vi "WriteOutSSH.vi"(11 "Write":string) -> (3 "text read":string)   [LabVIEW 2019]
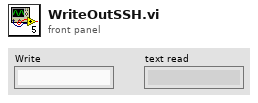
[diagram p1: front panel]
types:
  T1 = enum16{"init", "read", "write", "close", "wait", "reply"}
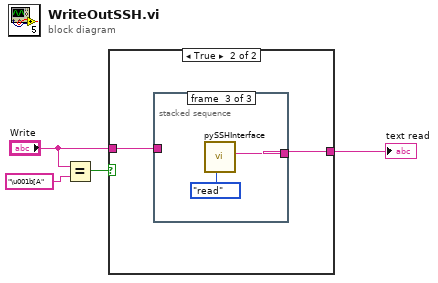
[diagram p0: block diagram]
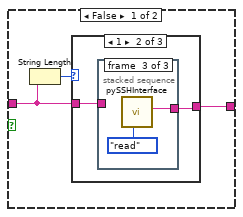
[diagram p2: hidden frame]
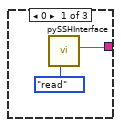
[diagram p3: hidden frame]
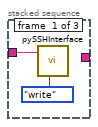
[diagram p4: hidden frame]
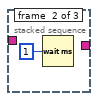
[diagram p5: hidden frame]
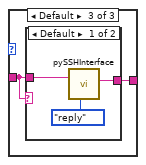
[diagram p6: hidden frame]
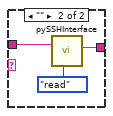
[diagram p7: hidden frame]
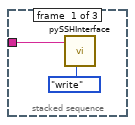
[diagram p8: hidden frame]
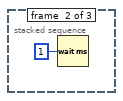
[diagram p9: hidden frame]
diagram:
  n1 = Equal?(x="Write", y="\u001b[A" ("string")) -> (x = y?=w1:bool)
  n2 = case shown="True" w1 {
    tunnel: [w6 w25] -> w4
    tunnel: "Write" -> [w5 w26]
    frame False {
      n3 = String Length(string=w5) -> (length=w7:i32)
      n4 = case shown="1" w7 {
        tunnel: [w8 w11 w18] -> w6
        tunnel: w5 -> [_ w10 w17]
        frame 0 {
          n5 = call <userlib>:"pySSHInterface.vi"("Task in"=T1."read") -> ("text read"=w8:string)  [unwired: 8 in, 2 out]
        }
        frame 1 {
          n6 = stacked-sequence {
            tunnel: [_ _ w15] -> w11
            tunnel: w10 -> [w12 _ _]
            frame #0 {
              n7 = call <userlib>:"pySSHInterface.vi"("Task in"=T1."write", "Text to write"=w12) -> ()  [unwired: 7 in, 3 out]
            }
            frame #1 {
              n8 = Wait (ms)(milliseconds to wait=u32 1) -> ()  [unwired: 1 out]
            }
            frame #2 {
              n9 = call <userlib>:"pySSHInterface.vi"("Task in"=T1."read") -> ("text read"=w15:string)  [unwired: 8 in, 2 out]
            }
          }
        }
        frame Default {
          n10 = case shown="Default" w17 {
            tunnel: w17 -> [w21 w24]
            tunnel: [w19 w22] -> w18
            frame Default {
              n11 = call <userlib>:"pySSHInterface.vi"("Task in"=T1."reply", "Text to write"=w21) -> ("text read"=w19:string)  [unwired: 7 in, 2 out]
            }
            frame "" {
              n12 = call <userlib>:"pySSHInterface.vi"("Task in"=T1."read", "Text to write"=w24) -> ("text read"=w22:string)  [unwired: 7 in, 2 out]
            }
          }
        }
      }
    }
    frame True {
      n13 = stacked-sequence {
        tunnel: [_ _ w30] -> w25
        tunnel: w26 -> [w27 _ _]
        frame #0 {
          n14 = call <userlib>:"pySSHInterface.vi"("Task in"=T1."write", "Text to write"=w27) -> ()  [unwired: 7 in, 3 out]
        }
        frame #1 {
          n15 = Wait (ms)(milliseconds to wait=u32 1) -> ()  [unwired: 1 out]
        }
        frame #2 {
          n16 = call <userlib>:"pySSHInterface.vi"("Task in"=T1."read") -> ("text read"=w30:string)  [unwired: 8 in, 2 out]
        }
      }
    }
  }
  "text read" <- w4
